vi "Ballard - Arinc-429 - Load Database.vi"(8 "error in (no error)":errorcluster, 11 "Node Ptr":u64 format="%.0x") -> (0 "error out":errorcluster)   [LabVIEW 2017, in "Ballard Arinc-429 System Explorer.lvlib"]
uses:
  Ballard Arinc-429 System Explorer.lvlib
  SubVIs/Create Sysdef Tree from DB Channel Clusters.vi
  SubVIs/Create Sysdef Tree Labels.vi
  SubVIs/Build Label Properties.vi
  Shared/Controls and Global/Global.vi
  <vilib>/NI Veristand/Custom Device API/Get Item Property (Path).vi
  SubVIs/Parse DB/Parse DB.vi
  <vilib>/NI Veristand/Custom Device API/NI VeriStand - Enable System Explorer Update Buffer.vi
  <vilib>/NI Veristand/Custom Device Tools/Custom Device Utility Library/NI VeriStand - Search for Item.vi
  <vilib>/NI Veristand/Custom Device Tools/Custom Device Utility Library/NI VeriStand - Search for Item by GUID.vi
  <vilib>/NI Veristand/Custom Device API/NI VeriStand - Add Custom Device Section.vi
  <vilib>/NI Veristand/Custom Device API/NI VeriStand - Add Custom Device Channel.vi
  SubVIs/Create Tx Word Description.vi
  <vilib>/NI Veristand/Custom Device API/NI VeriStand - Set Item Description.vi
  <vilib>/NI Veristand/Custom Device API/NI VeriStand - Commit System Explorer Update Buffer.vi
  SubVIs/Refresh DB/NI VeriStand - Visually Update the System Explorer Tree.vi
  <vilib>/NI Veristand/Custom Device API/Set Item Property (String).vi
  <vilib>/NI Veristand/Custom Device API/Set Item Property (Path).vi
  <vilib>/NI Veristand/Custom Device API/Custom Device API.lvlib
  Shared/Ballard Arinc-429 Shared.lvlib
  <vilib>/NI Veristand/Custom Device Tools/Custom Device Utility Library/Custom Device Utility Library.lvlib
panel:
  in  "Tag":string
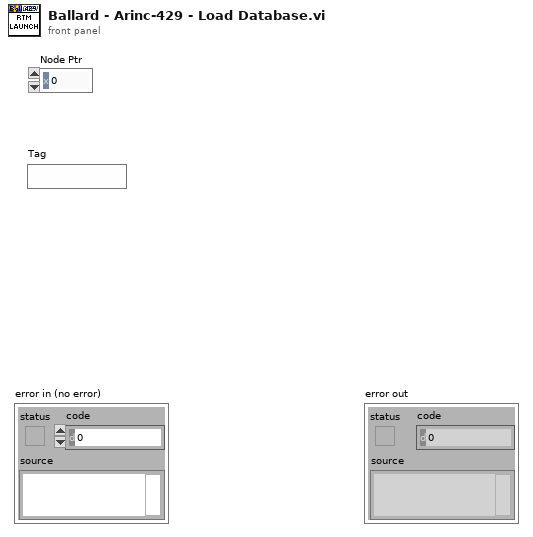
[diagram p1: front panel]
types:
  T1 = typedef "Custom Device API.lvlib/Custom Device Item Ref.ctl" = u64
  T2 = typedef "Ballard Arinc-429 System Explorer.lvlib/Refresh Match Settings.ctl" = cluster{"Ch by name?":bool, "Lbl by name?":bool}
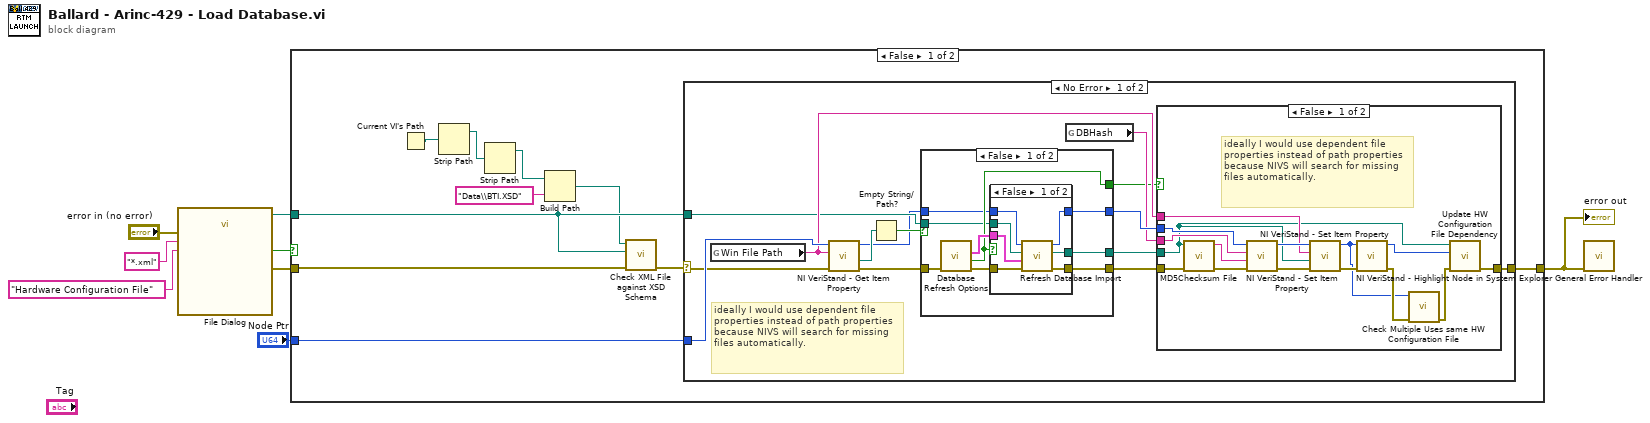
[diagram p0: block diagram]
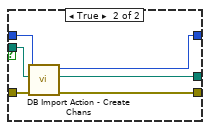
[diagram p4: hidden frame]
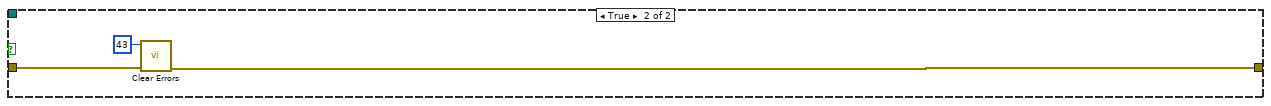
[diagram p6: hidden frame]
diagram:
  n1 = call "File Dialog"("error in"="error in (no error)", "pattern (all files)"="*.xml", "pattern label"="Hardware Configuration File") -> ("selected path"=w1:path, "cancelled"=w4:bool, "error out"=w3:errorcluster)  [unwired: 9 in, 1 out]
  n2 = case shown="False" w4 {
    tunnel: [w18 w75] -> w8
    tunnel: w3 -> [w15 w76]
    tunnel: "Node Ptr" -> [w17 _]
    tunnel: w1 -> [w14 _]
    frame False {
      n3 = Current VI's Path() -> (path=w11:path)
      n4 = Strip Path(path=w11) -> (stripped path=w12:path)  [unwired: 1 out]
      n5 = Strip Path(path=w12) -> (stripped path=w13:path)  [unwired: 1 out]
      n6 = Build Path(base path=w13, name or relative path="Data\\BTI.XSD") -> (appended path=w10:path)
      n7 = call "Check XML File against XSD Schema.vi"("error in (no error)"=w15, "XML Configuration File Path"=w14, "XML Schema File Path"=w10) -> ("error IO"=w16:errorcluster)  [unwired: 8 in]
      n8 = case shown="No Error" w16 {
        selector: w16 -> [w19 w74]
        tunnel: [w29 w74] -> w18
        tunnel: w17 -> [w27 _]
        tunnel: w14 -> [w23 _]
        frame No Error {
          # "ideally I would use dependent file properties instead of path properties because NIVS will search for missing files automatically."
          n9 = global read "Global.vi" "Win File Path"() -> (w26:string)
          n10 = call-poly <vilib>:"NI VeriStand - Get Item Property.vi"("error in (no error)"=w19, "Property Name"=w26, "Item Ref in"=w27) -> ("error out"=w20:errorcluster, "Value"=w24:path, "Item Ref out"=w21:T1)  [unwired: 5 in, 1 out]
          n11 = Empty String/Path?(string/path=w24) -> (empty?=w22:bool)
          n12 = case shown="False" w22 {
            tunnel: [w55 w73] -> w32
            tunnel: [w54 w72] -> w31
            tunnel: [w52 w71] -> w30
            tunnel: w20 -> [w57 w70]
            tunnel: [w51 _] -> w25
            tunnel: w23 -> [w50 w69]
            tunnel: w21 -> [w49 w68]
            frame False {
              n13 = call "Database Refresh Options.vi"("error in (no error)"=w57) -> ("error out"=w56:errorcluster, "Cancelled?"=w51:bool, "Refresh Settings"=w53:T2)  [unwired: 8 in]
              n14 = case shown="False" w51 {
                tunnel: w56 -> [w64 w67]
                tunnel: [w63 w67] -> w55
                tunnel: [w62 w65] -> w54
                tunnel: w50 -> [w59 w66]
                tunnel: w53 -> [w61 _]
                tunnel: [w60 w66] -> w52
                tunnel: w49 -> [w58 w65]
                frame False {
                  n15 = call "Refresh Database Import.vi"("error in (no error)"=w64, "Match settings"=w61, "DB"=w59, "Item Ref in"=w58) -> ("error out"=w63:errorcluster, "DB dup"=w60:path, "Item Ref dup"=w62:T1)  [unwired: 5 in]
                }
                frame True {
                }
              }
            }
            frame True {
              n16 = call "DB Import Action - Create Chans.vi"("error in (no error)"=w70, "selected path"=w69, "Node Ptr"=w68) -> ("error out"=w73:errorcluster, "selected path out"=w71:path, "Node Ptr dup"=w72:u64)  [unwired: 6 in]
            }
          }
          n17 = global read "Global.vi" "DBHash"() -> (w28:string)
          n18 = case shown="False" w25 {
            tunnel: w32 -> [w41 w48]
            tunnel: w31 -> [w47 _]
            tunnel: w30 -> [w37 _]
            tunnel: [w38 w48] -> w29
            tunnel: w28 -> [w43 _]
            tunnel: w26 -> [w42 _]
            frame False {
              # "ideally I would use dependent file properties instead of path properties because NIVS will search for missing files automatically."
              n19 = call <vilib>:"MD5Checksum File.vi"("error in (no error)"=w41, "Path"=w37) -> ("error out"=w40:errorcluster, "MD5 message-digest"=w39:string)  [unwired: 8 in]
              n20 = call-poly <vilib>:"NI VeriStand - Set Item Property.vi"("error in (no error)"=w40, "Value"=w39, "Property Name"=w43, "Item Ref in"=w47) -> ("error out"=w44:errorcluster, "Item Ref out"=w45:T1)  [unwired: 5 in, 1 out]
              n21 = call-poly <vilib>:"NI VeriStand - Set Item Property.vi"("error in (no error)"=w44, "Value"=w37, "Property Name"=w42, "Item Ref in"=w45) -> ("error out"=w46:errorcluster, "Item Ref out"=w33:T1)  [unwired: 5 in, 1 out]
              n22 = call <vilib>:"NI VeriStand - Highlight Node in System Explorer.vi"("error in (no error)"=w46, "Item Ref in"=w33) -> ("error out"=w35:errorcluster, "Node Ptr dup"=w36:T1)  [unwired: 8 in]
              n23 = call "Check Multiple Uses same HW Configuration File.vi"("error in (no error)"=w35, "Item Ref in"=w33) -> ("error out"=w34:errorcluster)  [unwired: 9 in]
              n24 = call "Update HW Configuration File Dependency.vi"("error in (no error)"=w34, "Node Ptr dup"=w36, "selected path in"=w37) -> ("error out"=w38:errorcluster)  [unwired: 8 in]
            }
            frame True {
            }
          }
        }
        frame Error {
        }
      }
    }
    frame True {
      n25 = call <vilib>:"Clear Errors.vi"("error in (no error)"=w76, "specific error code to clear (0: all)"=43) -> ("error out"=w75:errorcluster)  [unwired: 4 in, 1 out]
    }
  }
  "error out" <- w8
  n26 = call <vilib>:"General Error Handler.vi"("error in (no error)"=w8) -> ()  [unwired: 10 in, 5 out]
